vi "Update Missed Samples.vi"(8 "error in (no error)":errorcluster, 9 "Samples Missed":u64, 11 "Waveform Log in":refnum<class "Waveform Log.lvclass">) -> (0 "error out":errorcluster, 3 "Waveform Log out":refnum<class "Waveform Log.lvclass">)   [LabVIEW 2015, in "Waveform Data Logger Engine.lvlib" / "Waveform Log.lvclass"]
uses:
  Waveform Log.lvclass
  Waveform Log.lvclass/Waveform Log.ctl
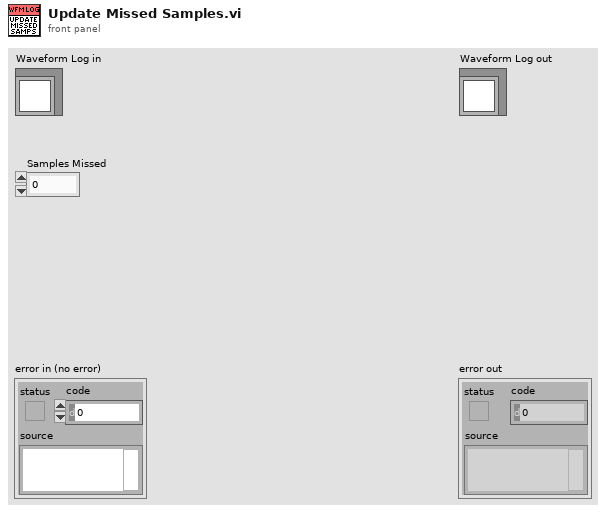
[diagram p1: front panel]
types:
  T1 = typedef "Waveform Data Logger Engine.lvlib/Waveform Log.lvclass/Log Instance.ctl" = cluster{"Segmented Log":refnum<data-value>, "Log Waveforms":T2[], "Log Start":timestamp, "Log Stop":timestamp, "Start Trigger Time":timestamp, "Stop Trigger Time":timestamp, "Time of Last Write":timestamp, "Timeout":dbl, "Stop cmd received":bool}
  T2 = typedef "Waveform Data Logger Engine.lvlib/Waveform Log.lvclass/Log Instance Waveform.ctl" = cluster{"Wfm Info":T3, "Count / Instance":i32, "Previous Segment":u64, "Wfm Complete?":bool, "Last Sample Logged":timestamp, "Data Logged":bool, "Log segmented":bool}
  T3 = typedef "Waveform Data Logger Engine.lvlib/Waveform Log.lvclass/Waveform Information.ctl" = cluster{"Name":string, "Wfm Data Type":T4, "Decimation":u32}
  T4 = typedef "Waveform Data Logger Engine.lvlib/Waveform Log.lvclass/Waveform Data Type.ctl" = enum16{"Double", "ComplexDouble"}
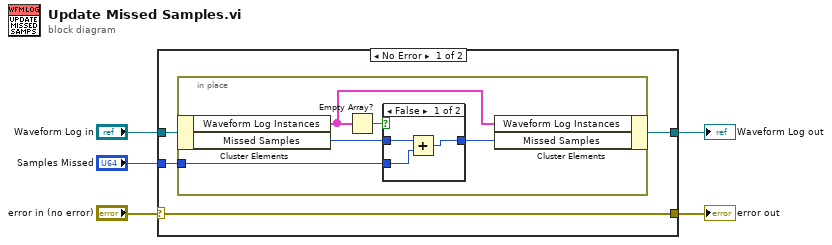
[diagram p0: block diagram]
diagram:
  n1 = case shown="No Error" "error in (no error)" {
    selector: "error in (no error)" -> [w9 w20]
    tunnel: [w9 w20] -> w4
    tunnel: [w6 w19] -> w2
    tunnel: "Waveform Log in" -> [w8 w19]
    tunnel: "Samples Missed" -> [w7 _]
    frame No Error {
      n2 = in-place {
        in-place-border: w7 -> [w13]
        n3 = in-place-cluster #1(w8) -> ("Waveform Log Instances"=w10:T1[], "Missed Samples"=w14:u64)
        n4 = Empty Array?(array=w10) -> (empty?=w11:bool)
        n5 = case shown="False" w11 {
          tunnel: w14 -> [w17 w18]
          tunnel: w13 -> [w16 _]
          tunnel: [w15 w18] -> w12
          frame False {
            n6 = Add(x=w17, y=w16) -> (x+y=w15:u64)
          }
          frame True {
          }
        }
        n7 = in-place-cluster #1("Waveform Log Instances"=w10, "Missed Samples"=w12) -> (w6:refnum<class "Waveform Log.lvclass">)
      }
    }
    frame Error {
    }
  }
  "error out" <- w4
  "Waveform Log out" <- w2
